vi "aceleration_sub.vi"(7 "acceleration_pre":fxp<+/-,20,9>, 8 "ticks_m_pre":u32, 9 "ticks":u32, 10 "count_pre":i32, 11 "count":i32) -> (0 "ticks_m":u32, 3 "acceleration (mm/s2)":fxp<+/-,20,9>)   [LabVIEW 2014]
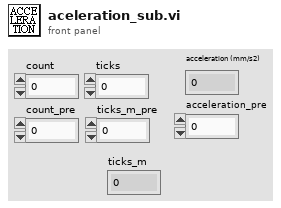
[diagram p1: front panel]
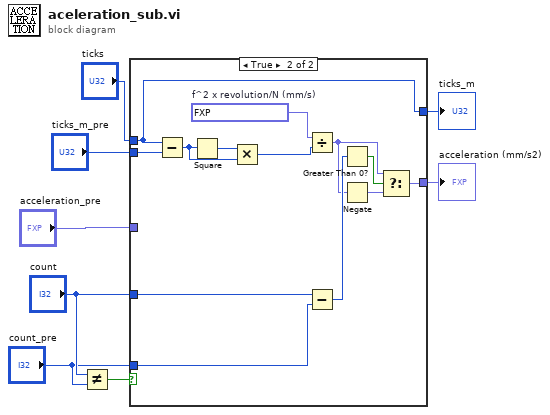
[diagram p0: block diagram]
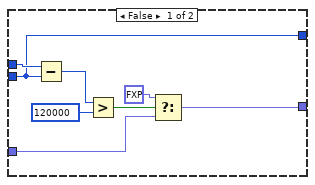
[diagram p2: hidden frame]
diagram:
  n1 = Not Equal?(x="count", y="count_pre") -> (x != y?=w8:bool)
  n2 = case shown="True" w8 {
    tunnel: "ticks" -> [w16 w26]
    tunnel: "count" -> [_ w29]
    tunnel: "count_pre" -> [_ w28]
    tunnel: [w15 w26] -> w1
    tunnel: "ticks_m_pre" -> [w15 w25]
    tunnel: [w11 w20] -> w5
    tunnel: "acceleration_pre" -> [w12 _]
    frame False {
      n3 = Subtract(x=w16, y=w15) -> (x-y=w14:u32)
      n4 = Greater?(x=w14, y=u32 120000) -> (0:w13:bool)
      n5 = Select(t=fxp<+/-,20,9> 0.0, s=w13, f=w12) -> (s? t:f=w11:fxp<+/-,20,9>)
    }
    frame True {
      w22 = fxp<+,41,41> 1600000000000.0  # f^2 x revolution/N (mm/s)
      n6 = Subtract(x=w26, y=w25) -> (x-y=w18:u32)
      n7 = Square(x=w18) -> (x^2=w19:u32)
      n8 = Multiply(x=w19, y=w18) -> (x*y=w17:u32)
      n9 = Divide(x=w22, y=w17) -> (x/y=w23:fxp<+/-,20,9>)
      n10 = Subtract(x=w29, y=w28) -> (x-y=w27:i32)
      n11 = Greater Than 0?(x=w27) -> (x > 0?=w21:bool)
      n12 = Negate(x=w23) -> (-x=w24:fxp<+/-,20,9>)
      n13 = Select(t=w23, s=w21, f=w24) -> (s? t:f=w20:fxp<+/-,20,9>)
    }
  }
  "acceleration (mm/s2)" <- w5
  "ticks_m" <- w1
